vi "DequeVa.vi"(8 "エラー入力（エラーなし）":errorcluster, 9 "タイムアウト（ms）（-1）":i32=-1, 11 "queVariant":refnum<queue>) -> (0 "エラー出力":errorcluster, 1 "timed out?":bool, 2 "バリアント":variant, 3 "queVariant(copy)":refnum<queue>, 4 "コマンド":string)   [LabVIEW 2016]
uses:
  Event/Ctl/EventVariantData.ctl
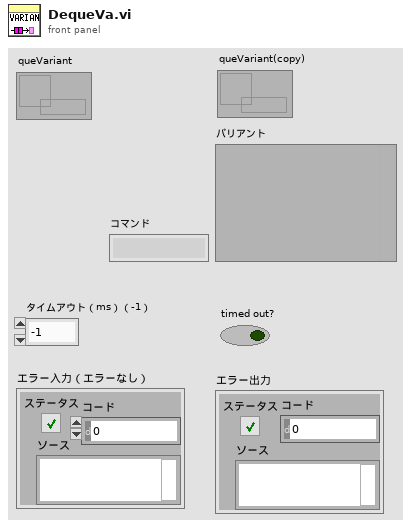
[diagram p1: front panel]
types:
  T1 = typedef "EventVariantData.ctl" = cluster{"コマンド":string, "バリアント":variant}
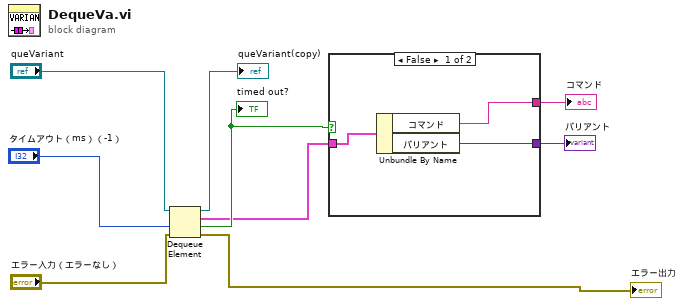
[diagram p0: block diagram]
diagram:
  n1 = Dequeue Element(queue="queVariant", timeout in ms (-1)="タイムアウト（ms）（-1）", error in (no error)="エラー入力（エラーなし）") -> (queue out=→"queVariant(copy)":refnum<queue>, element=w5:T1, timed out?=w8:bool, error out=→"エラー出力":errorcluster)
  "timed out?" <- w8
  n2 = case shown="FALSE" w8 {
    tunnel: [w10 _] -> w7
    tunnel: [w11 _] -> w6
    tunnel: w5 -> [w12 _]
    frame False {
      n3 = Unbundle By Name(w12) -> ("コマンド"=w10:string, "バリアント"=w11:variant)
    }
    frame True {
    }
  }
  "コマンド" <- w7
  "バリアント" <- w6
